vi "Alliance_ID.vi"() -> ()   [LabVIEW 2016]
panel:
  out "Alliance":dbl
  out "Position":dbl
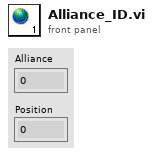
[diagram p1: front panel]
diagram:
